vi "RunTest - Select Device.vi"(8 "error in (no error)":errorcluster, 11 "Item Names":string[](array[string])) -> (0 "error out":errorcluster, 2 "Cancel":bool=TRUE, 3 "Device":string)   [LabVIEW 2019]
panel:
  in  "Cancel":bool
  in  "Ok":bool
  in  "Device":i32(listbox)
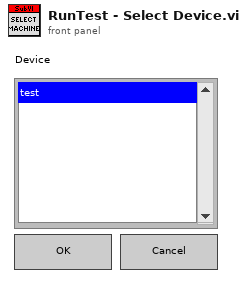
[diagram p1: front panel]
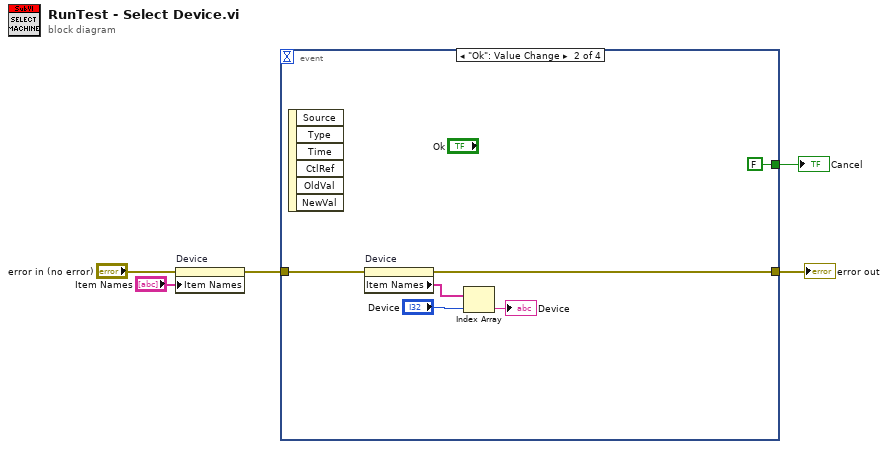
[diagram p0: block diagram]
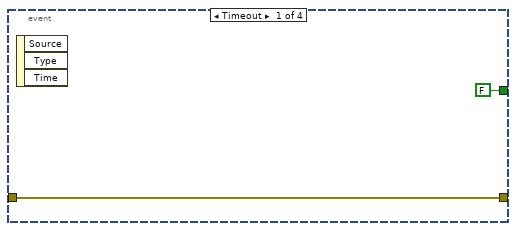
[diagram p2: hidden frame]
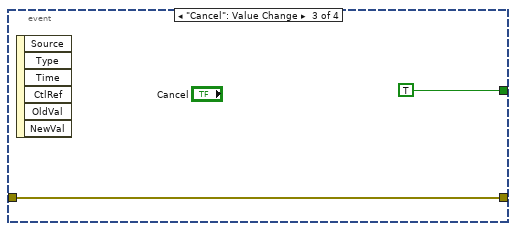
[diagram p3: hidden frame]
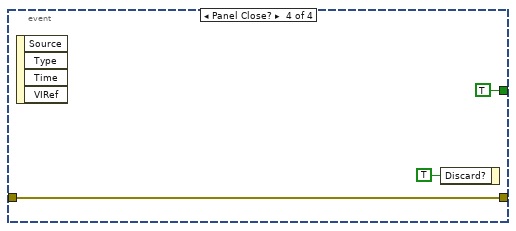
[diagram p4: hidden frame]
diagram:
  n1 = property on="Device" class="LstBox (strict)"(error in="error in (no error)", "Item Names"="Item Names") -> (error out=w4:errorcluster)  [unwired: 1 in, 1 out]
  n2 = event shown="[1] \"Ok\": Value Change" {
    selector: _ -> [_ _ _ _]
    dyn-events: _ -> [_ _ _ _]
    timeout: _ -> [_ _ _ _]
    tunnel: w4 -> [w7 w13 w15 w17]
    tunnel: [w7 w10 w15 w17] -> w2
    tunnel: [FALSE FALSE TRUE TRUE] -> w1
    event Timeout {
      n3 = event-data() -> ()  [unwired: 1 in, 3 out]
    }
    event "Ok": Value Change {
      n4 = event-data() -> ()  [unwired: 1 in, 6 out]
      n5 = property on="Device" class="LstBox (strict)"(error in=w13) -> (error out=w10:errorcluster, "Item Names"=w12:string[])  [unwired: 1 in, 1 out]
      n6 = Index Array(array=w12, index="Device") -> (element=→"Device":string)
    }
    event "Cancel": Value Change {
      n7 = event-data() -> ()  [unwired: 1 in, 6 out]
    }
    event Panel Close? {
      n8 = event-data() -> ()  [unwired: 1 in, 4 out]
      n9 = event-data("Discard?"=TRUE) -> ()  [unwired: 1 in, 1 out]
    }
  }
  "error out" <- w2
  "Cancel" <- w1
